vi "Set Range.vi"(8 "error in":errorcluster, 10 "Range":T1={"Input Ranging Mode (Auto)"=enum."AUTO", "Input Input Type (Internal)"=1, "Input Selection (CH1)"=enum."CH1", "Input Connection (Main) "=0, "Input Coupling (Internal)"=enum."AC+DC", "Input Shunt Value (0,02)"=0.02, "Input Voltage Scale factor (1)"=1.0} {"Input Voltage Scale factor (1)" min=0.0 max=100000.0 step=0.001; "Input Shunt Value (0,02)" min=1e-06 max=10.0 step=1e-06; "Input Connection (Main)" items=["MAIN", "SECONDARY", "DIFFERENTIAL"]; "Input Input Type (Internal)" items=["DISABLED", "INTERNAL", "EXTERNAL SHUNT"]}) -> (0 "error out":errorcluster)   [LabVIEW 2025, in "N4L_PSM3750_Interface.lvlib"]
doc: "Sets the measurement range.\n\n_____\nCreated using DQMH Framework: Event Scripter 7.1.0.1503."
uses:
  N4L_PSM3750_Interface.lvlib
  Range Config--cluster.ctl
  Set Range Argument--cluster.ctl
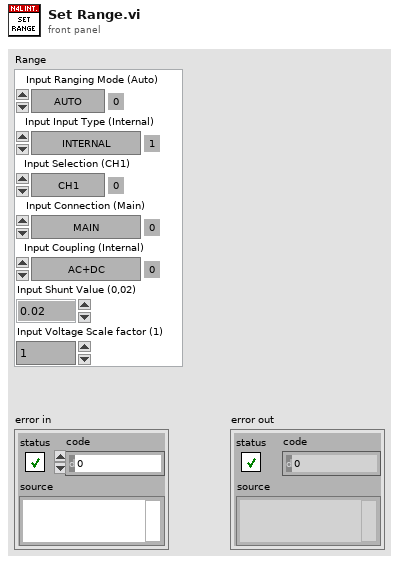
[diagram p1: front panel]
types:
  T1 = typedef "N4L_PSM3750_Interface.lvlib/Range Config--cluster.ctl" = cluster{"Input Ranging Mode (Auto)":enum16{"AUTO", "UPAUTO", "1mV", "3mV", "10mV", "30mV", "100mV", "300mV", "1V", "3V", "10V"}, "Input Input Type (Internal)":u16, "Input Selection (CH1)":enum16{"CH1", "CH2"}, "Input Connection (Main) ":u16, "Input Coupling (Internal)":enum16{"AC+DC", "AC"}, "Input Shunt Value (0,02)":dbl, "Input Voltage Scale factor (1)":dbl}
  T2 = typedef "N4L_PSM3750_Interface.lvlib/Set Range Argument--cluster.ctl" = cluster{"Range":T1}
  T3 = typedef "N4L_PSM3750_Interface.lvlib/Request Events--cluster.ctl" = cluster{"Stop Module":refnum<user-event>, "Show Panel":refnum<user-event>, "Hide Panel":refnum<user-event>, "Get Module Execution Status":refnum<user-event>, "Show Diagram":refnum<user-event>, "Change Panel":refnum<user-event>, "Initialise N4L Connection":refnum<user-event>, "Close N4L Connection":refnum<user-event>, "Reset N4L Instrument":refnum<user-event>, "Set Generator Configuration":refnum<user-event>, "Set Generator Output":refnum<user-event>, "Set Range":refnum<user-event>, "Set Trim Configuration":refnum<user-event>}
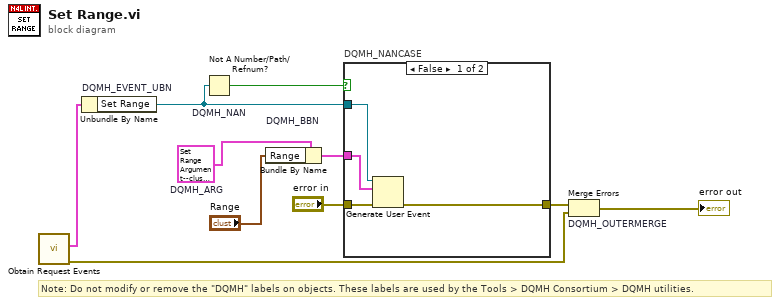
[diagram p0: block diagram]
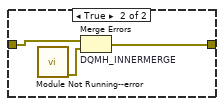
[diagram p2: hidden frame]
diagram:
  w4 = T2 {"Range"={"Input Ranging Mode (Auto)"=enum."AUTO", "Input Input Type (Internal)"=1, "Input Selection (CH1)"=enum."CH1", "Input Connection (Main) "=0, "Input Coupling (Internal)"=enum."AC+DC", "Input Shunt Value (0,02)"=0.02, "Input Voltage Scale factor (1)"=1.0}}  # DQMH_ARG
  # "Note: Do not modify or remove the \"DQMH\" labels on objects. These labels are used by the Tools > DQMH Consortium > DQMH utilities."
  n1 = call "Obtain Request Events.vi"() -> ("error out"=w2:errorcluster, "N4L_PSM3750_Interface Request Events"=w1:T3)  [unwired: 10 in]
  n2 = Unbundle By Name "DQMH_EVENT_UBN"(w1) -> ("Set Range"=w6:refnum<user-event>)
  n3 = Not A Number/Path/Refnum? "DQMH_NAN"(number/path/refnum=w6) -> (NaN/Path/Refnum?=w7:bool)
  n4 = Bundle By Name "DQMH_BBN"(cluster=w4, "Range"="Range") -> (w8:T2)
  n5 = case "DQMH_NANCASE" shown="False" w7 {
    tunnel: "error in" -> [w14 w17]
    tunnel: [w13 w16] -> w5
    tunnel: w6 -> [w12 _]
    tunnel: w8 -> [w11 _]
    frame False {
      n6 = Generate User Event(user event=w12, event data cluster=w11, error in=w14) -> (error out=w13:errorcluster)  [unwired: 1 in, 1 out]
    }
    frame True {
      n7 = call "Module Not Running--error.vi"() -> ("error out"=w15:errorcluster)  [unwired: 11 in]
      n8 = Merge Errors "DQMH_INNERMERGE"(w17, w15) -> (w16:errorcluster)
    }
  }
  n9 = Merge Errors "DQMH_OUTERMERGE"(w5, w2) -> (→"error out":errorcluster)
